vi "MBtcp-ReadAny.vi"(0 "IP Address":string caption="IP Address(:Port(502)) (from Port Name)", 2 "Ch Name":string, 3 "Slave ID":u8=255 format="%.0x", 5 "Register":u16 caption="Register (from Ch.)", 7 "DataType(:RegisterType)":string, 11 "Error In":errorcluster) -> (4 "Value":dbl, 6 "Read At":timestamp, 15 "error out":errorcluster)   [LabVIEW 2020]
uses:
  RegisterTypes.ctl
panel:
  out "RegisterType":T1="Input" caption="RegisterType (from Comments)"
  out "Data type":string(combo) caption="Data type (from Comments)"
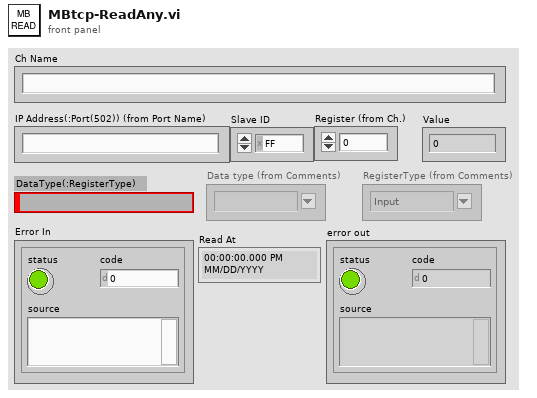
[diagram p1: front panel]
types:
  T1 = typedef "RegisterTypes.ctl" = string
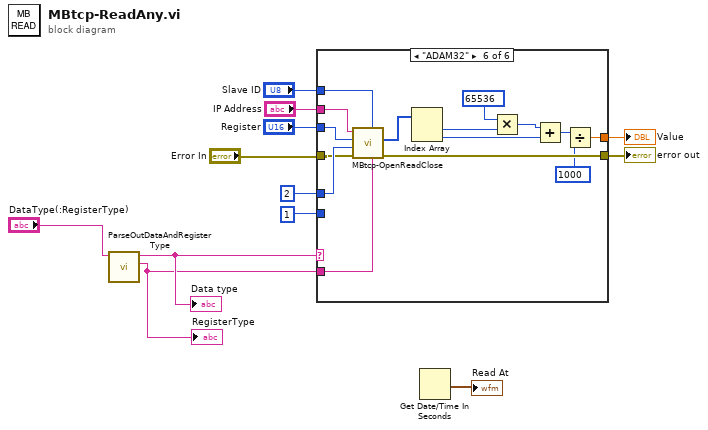
[diagram p0: block diagram]
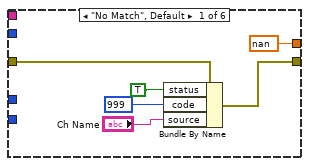
[diagram p2: hidden frame]
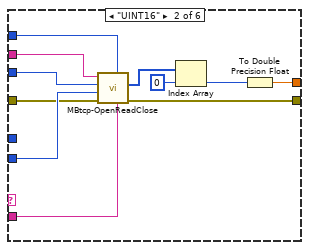
[diagram p3: hidden frame]
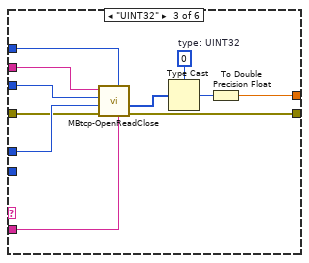
[diagram p4: hidden frame]
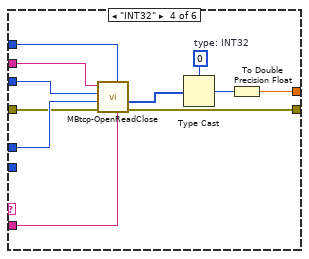
[diagram p5: hidden frame]
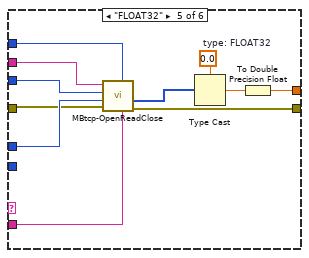
[diagram p6: hidden frame]
diagram:
  n1 = call "ParseOutDataAndRegisterType.vi"("DataType(:RegisterType) in"="DataType(:RegisterType)") -> ("RegisterType"=w1:string, "DataType"=w2:string)  [unwired: 9 in]
  "Data type" <- w2
  "RegisterType" <- w1
  n2 = case shown="\"ADAM32\"" w2 {
    tunnel: [w18 w26 w34 w48 w59 w77] -> w10
    tunnel: [nan w28 w39 w50 w61 w66] -> w12
    tunnel: u16 2 ("Num Registers to read") -> [_ _ w37 w44 w55 w74]
    tunnel: "Register" -> [_ w23 w36 w45 w56 w75]
    tunnel: "IP Address" -> [_ w24 w35 w46 w58 w76]
    tunnel: u16 1 ("Num Registers to read") -> [_ w22 _ _ _ _]
    tunnel: "Error In" -> [w13 w21 w32 w43 w54 w73]
    tunnel: "Slave ID" -> [_ w20 w31 w42 w53 w72]
    tunnel: w1 -> [_ w19 w30 w41 w52 w71]
    frame "No Match", Default {
      n3 = Bundle By Name(cluster=w13, "status"=TRUE, "code"=999, "source"="Ch Name") -> (w18:errorcluster)
    }
    frame "UINT16" {
      n4 = call "MBtcp-OpenReadClose.vi"("RegisterType"=w19, "Slave ID"=w20, "error in (no error)"=w21, "nRegisters"=w22, "RegisterAddr"=w23, "IP Address(:port)"=w24) -> ("error out"=w26:errorcluster, "16bitValues"=w25:u16[])  [unwired: 3 in, 1 out]
      n5 = Index Array(array=w25, index=0) -> (element=w29:u16)
      n6 = To Double Precision Float(number=w29) -> (double precision float=w28:dbl)
    }
    frame "UINT32" {
      w38 = u32 0  # type: UINT32
      n7 = call "MBtcp-OpenReadClose.vi"("RegisterType"=w30, "Slave ID"=w31, "error in (no error)"=w32, "nRegisters"=w37, "RegisterAddr"=w36, "IP Address(:port)"=w35) -> ("error out"=w34:errorcluster, "32bitValues"=w33:u32[])  [unwired: 3 in, 1 out]
      n8 = Type Cast(type=w38, x=w33) -> (*(type *) &x=w40:u32)
      n9 = To Double Precision Float(number=w40) -> (double precision float=w39:dbl)
    }
    frame "INT32" {
      w49 = 0  # type: INT32
      n10 = call "MBtcp-OpenReadClose.vi"("RegisterType"=w41, "Slave ID"=w42, "error in (no error)"=w43, "nRegisters"=w44, "RegisterAddr"=w45, "IP Address(:port)"=w46) -> ("error out"=w48:errorcluster, "32bitValues"=w47:u32[])  [unwired: 3 in, 1 out]
      n11 = Type Cast(type=w49, x=w47) -> (*(type *) &x=w51:i32)
      n12 = To Double Precision Float(number=w51) -> (double precision float=w50:dbl)
    }
    frame "FLOAT32" {
      w60 = sgl 0.0  # type: FLOAT32
      n13 = call "MBtcp-OpenReadClose.vi"("RegisterType"=w52, "Slave ID"=w53, "error in (no error)"=w54, "nRegisters"=w55, "RegisterAddr"=w56, "IP Address(:port)"=w58) -> ("error out"=w59:errorcluster, "32bitValues"=w57:u32[])  [unwired: 3 in, 1 out]
      n14 = Type Cast(type=w60, x=w57) -> (*(type *) &x=w62:sgl)
      n15 = To Double Precision Float(number=w62) -> (double precision float=w61:dbl)
    }
    frame "ADAM32" {
      n16 = call "MBtcp-OpenReadClose.vi"("RegisterType"=w71, "Slave ID"=w72, "error in (no error)"=w73, "nRegisters"=w74, "RegisterAddr"=w75, "IP Address(:port)"=w76) -> ("error out"=w77:errorcluster, "16bitValues"=w65:u16[])  [unwired: 3 in, 1 out]
      n17 = Index Array(array=w65) -> (element #1=w63:u16, element #2=w64:u16)  [unwired: 2 in]
      n18 = Multiply(x=65536, y=w63) -> (x*y=w68:i32)
      n19 = Add(x=w68, y=w64) -> (x+y=w69:i32)
      n20 = Divide(x=w69, y=1000) -> (x/y=w66:dbl)
    }
  }
  "Value" <- w12
  "error out" <- w10
  n21 = Get Date/Time In Seconds() -> (seconds since 1Jan1904=→"Read At":timestamp)
